vi "qp_AS lagrange multipliers.vi"(10 "Qx+c":dbl[](array[numeric]), 11 "A working set":T1) -> (3 "lagrange multipliers":dbl[](array[numeric]))   [LabVIEW 2017, in "NI_Gmath.lvlib"]
uses:
  <vilib>/gmath/NI_Gmath.lvlib
  <vilib>/Analysis/Matrix/Datatypes/RealMatrix.ctl
  <vilib>/Analysis/7linalg.llb/Solve Linear Equations (single right hand).vi
  <vilib>/Analysis/baseanly.llb/Solve Linear Equations By Cholesky.vi
  <vilib>/Analysis/baseanly.llb/Real Matrix to Compact Array.vi
  <vilib>/Analysis/baseanly.llb/Real Compact Tri-Matrix Linear Eqs.vi
  <vilib>/Analysis/7linalg.llb/Solve Linear Eqs (General).vi
  <vilib>/Analysis/7linalg.llb/Solve Linear Eqs (Gen, single right hand).vi
  <vilib>/Analysis/NI_AALPro.lvlib
  <vilib>/Analysis/Matrix/NI_Matrix.lvlib
panel:
  out "error":i32
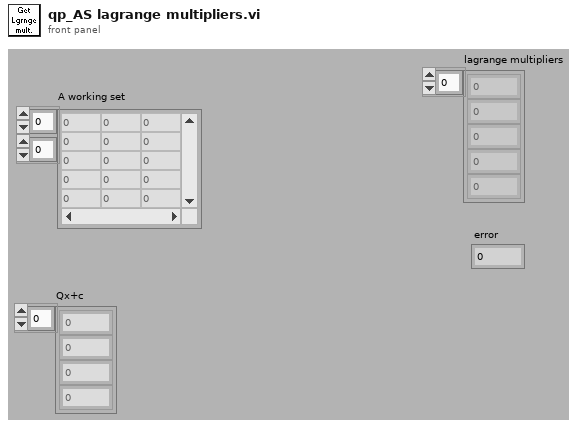
[diagram p1: front panel]
types:
  T1 = typedef "NI_Matrix.lvlib/RealMatrix.ctl" = dbl[][]
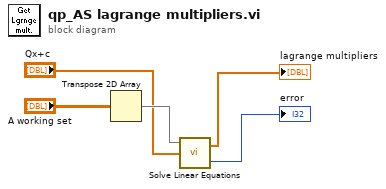
[diagram p0: block diagram]
diagram:
  n1 = Transpose 2D Array(2D array="A working set") -> (transposed array=w4:T1)
  n2 = call-poly <vilib>:"Solve Linear Equations.vi"("Known Vector"="Qx+c", "Input Matrix"=w4) -> ("error"=→"error":i32, "Solution Vector"=→"lagrange multipliers":dbl[])  [unwired: 1 in]
